vi "ReadStartupBehavior.vi"(8 "error in (no error)":errorcluster, 11 "SMO in":refnum<class "SMO.lvclass">) -> (0 "error out":errorcluster, 2 "Behavior":T1, 3 "SMO out":refnum<class "SMO.lvclass">)   [LabVIEW 2013, in "SMO.lvclass"]
uses:
  SMO.lvclass
  Support/Attribute.StartupBehavior/ProcessStartupBehavior.ctl
  Support/Attribute.StartupBehavior/Attribute.StartupBehavior.lvclass
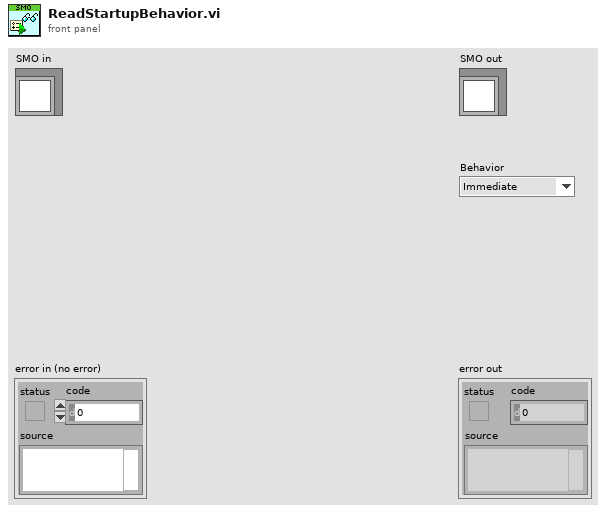
[diagram p1: front panel]
types:
  T1 = typedef "SMOAttributes.lvlib/Attribute.StartupBehavior.lvclass/ProcessStartupBehavior.ctl" = enum16{"Immediate", "First Call", "Never"}
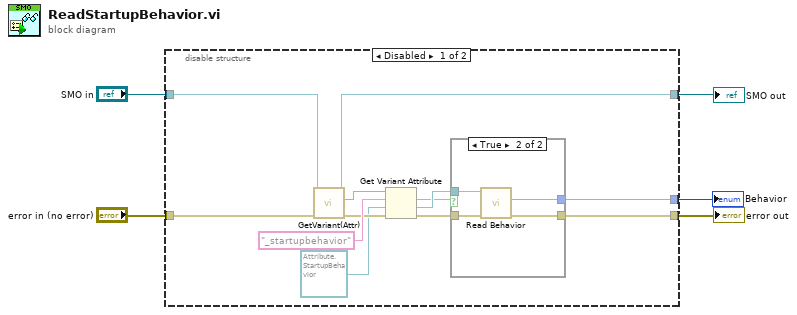
[diagram p0: block diagram]
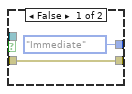
[diagram p2: hidden frame]
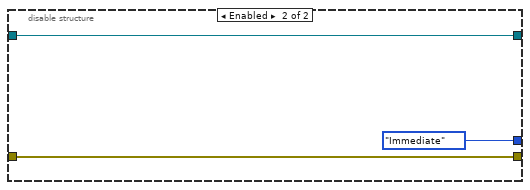
[diagram p3: hidden frame]
diagram:
  n1 = disable-structure shown="Disabled" {
    disable-tunnel: "SMO in" -> [w13 w25]
    disable-tunnel: "error in (no error)" -> [w14 w24]
    disable-tunnel: [w12 w25] -> w3
    disable-tunnel: [w8 w24] -> w2
    disable-tunnel: [w7 ProcessStartupBehavior."Immediate" ("t")] -> w1
    frame Disabled {
      n2 = call "GetVariant(Attr).vi"("error in (no error)"=w14, "SMO in"=w13) -> ("error out"=w15:errorcluster, "[Attributes]"=w17:variant, "SMO out"=w12:refnum<class "SMO.lvclass">)  [unwired: 7 in]
      n3 = Get Variant Attribute(Variant=w17, name="_startupbehavior", default value (empty Variant)=refnum<class "Attribute.StartupBehavior.lvclass"> refnum ("Attribute.StartupBehavior.lvclass"), error in=w15) -> (found=w6:bool, value=w10:refnum<class "Attribute.StartupBehavior.lvclass">, error out=w9:errorcluster)  [unwired: 1 out]
      n4 = case shown="True" w6 {
        tunnel: w10 -> [_ w23]
        tunnel: w9 -> [w19 w22]
        tunnel: [w19 w21] -> w8
        tunnel: [ProcessStartupBehavior."Immediate" ("Behavior") w20] -> w7
        frame False {
        }
        frame True {
          n5 = call "Read Behavior.vi"("error in (no error)"=w22, "Attribute.StartupBehavior in"=w23) -> ("error out"=w21:errorcluster, "Behavior"=w20:T1)  [unwired: 7 in, 1 out]
        }
      }
    }
    frame Enabled {
    }
  }
  "error out" <- w2
  "SMO out" <- w3
  "Behavior" <- w1
